vi "Save Parameter.vi"(7 "En Pop up":bool, 8 "Para In":dbl[](array[numeric]), 9 "Name":string[](array[string]), 11 "Save Path":path) -> (3 "dup path":path)   [LabVIEW 2017]
uses:
  <vilib>/Utility/file.llb/Write Delimited Spreadsheet (string).vi
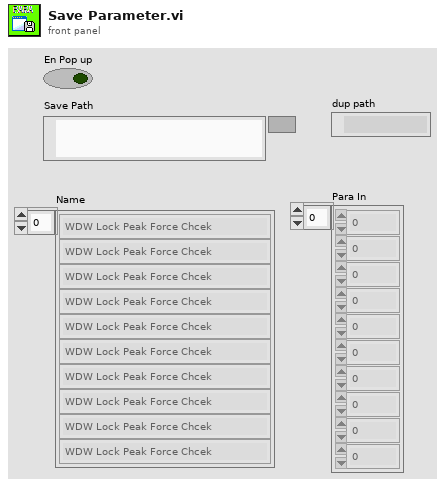
[diagram p1: front panel]
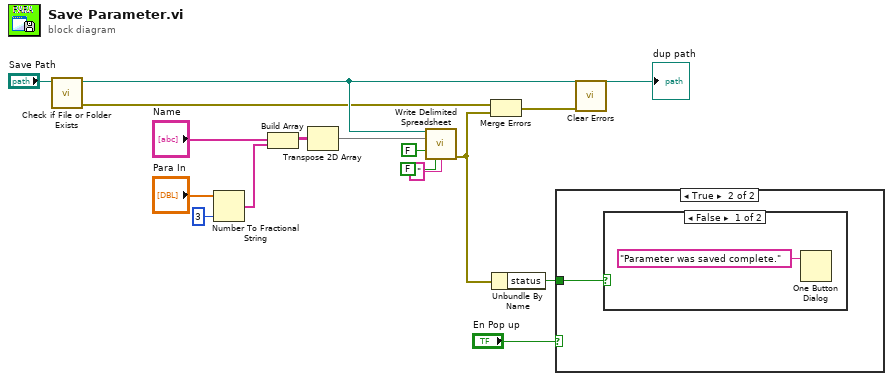
[diagram p0: block diagram]
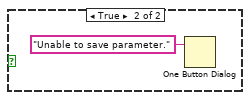
[diagram p3: hidden frame]
diagram:
  n1 = call <vilib>:"Check if File or Folder Exists.vi"("path"="Save Path") -> ("error out"=w2:errorcluster, "dup path"=w16:path)  [unwired: 8 in, 1 out]
  "dup path" <- w16
  n2 = Number To Fractional String(number="Para In", precision (6)=i16 3) -> (F-format string=w10:string[])  [unwired: 2 in]
  n3 = Build Array("Name", w10) -> (w11:string[][])
  n4 = Transpose 2D Array(2D array=w11) -> (transposed array=w6:string[][])
  n5 = call-poly <vilib>:"Write Delimited Spreadsheet.vi"("file path (dialog if empty)"=w16, "2D data"=w6, "append to file? (new file:F)"=FALSE, "transpose? (no:F)"=FALSE, "delimiter (\\t)"="," ("delimiter (\\t)")) -> ("error out"=w4:errorcluster)  [unwired: 9 in, 1 out]
  n6 = Merge Errors(w2, w4) -> (w3:errorcluster)
  n7 = Unbundle By Name(w4) -> ("status"=w5:bool)
  n8 = case shown="True" "En Pop up" {
    tunnel: w5 -> [_ w17]
    frame False {
    }
    frame True {
      n9 = case shown="False" w17 {
        frame False {
          n10 = One Button Dialog(message="Parameter was saved complete.") -> ()  [unwired: 1 in, 1 out]
        }
        frame True {
          n11 = One Button Dialog(message="Unable to save parameter.") -> ()  [unwired: 1 in, 1 out]
        }
      }
    }
  }
  n12 = call <vilib>:"Clear Errors.vi"("error in (no error)"=w3) -> ()  [unwired: 5 in, 2 out]
